vi "Teleop.vi"(10 "Match Info":T1={"Autonomous Elapsed Seconds"=0.0, "TeleOp Elapsed Seconds"=43.06, "Disabled Elapsed Seconds"=6.912, "Visited Autonomous"=FALSE, "Visited TeleOp"=TRUE, "Visited Disabled"=TRUE, "Autonomous Settings"={"Autonomous Style"=enum."Independent", "VI Refnum"=refnum}}, 11 "Call Context":T2=enum."Stop") -> ()   [LabVIEW 2019]
doc: "This VI is called for each TeleOp packet received from the DS where the robot is not disabled. It is often used to read from the joysticks and update I/O or to update setpoints for timed control loops. It should complete and return within 20 milliseconds or it may miss DS packets."
uses:
  <vilib>/Rock Robotics/WPI/DriverStation/WPI_DriverStationDerivedRobotMode.ctl
  <vilib>/Rock Robotics/WPI/DriverStation/WPI_DriverStationMatch Info.ctl
  <vilib>/Rock Robotics/WPI/Solenoid/WPI_SolenoidValue.ctl
  Global Data.vi
  <vilib>/Rock Robotics/Network Tables/NT Write Number.vi
  Refnums.vi
  <vilib>/Rock Robotics/Network Tables/NT Write Numeric Array.vi
  <vilib>/Rock Robotics/Network Tables/NT Write Boolean Array.vi
  Buttons.vi
  <vilib>/Rock Robotics/WPI/Solenoid/WPI_SolenoidSetEnum.vi
  <vilib>/Rock Robotics/WPI/ThirdParty/Phoenix-LabVIEW/Motor Controller/Controls/CTRE_Phoenix_MotorControl_ControlMode.ctl
  <vilib>/Rock Robotics/WPI/ThirdParty/Phoenix-LabVIEW/Motor Controller/Get/CTRE_Phoenix_MotorController_GetQuadratureData.vi
panel:
  in  "f":enum16{"Spin-Up", "Shoot", "Stop"}(ring)
  in  "AngleSet":dbl
  out "Angle Position":dbl=4.0
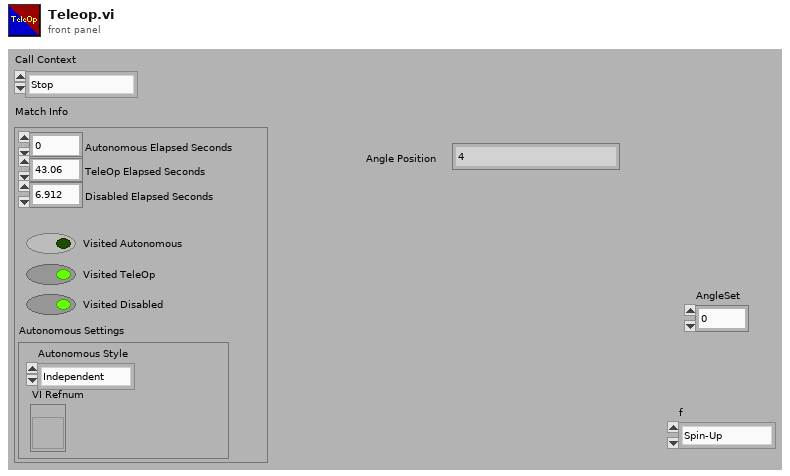
[diagram p1: front panel]
types:
  T1 = typedef "WPI_DriverStationMatch Info.ctl" = cluster{"Autonomous Elapsed Seconds":dbl, "TeleOp Elapsed Seconds":dbl, "Disabled Elapsed Seconds":dbl, "Visited Autonomous":bool, "Visited TeleOp":bool, "Visited Disabled":bool, "Autonomous Settings":cluster{"Autonomous Style":enum16{"Iterative", "Independent"}, "VI Refnum":refnum<vi>}}
  T2 = typedef "WPI_DriverStationDerivedRobotMode.ctl" = enum16{"Init", "Execute", "Stop"}
  T3 = typedef "WPI_SolenoidValue.ctl" = enum16{"Off", "On", "Forward", "Reverse"}
  T4 = typedef "WPI_JoystickDevRef.ctl" = cluster{"Device":T5}
  T5 = typedef "WPI_JoystickDeviceEnum.ctl" = enum16{"USB 0", "USB 1", "USB 2", "USB 3", "USB 4", "USB 5"}
  T6 = cluster{"Align Turret":i32, "Turret Right":i32, "TODO 1":i32, "Turret Left":i32, "Jump Intake":i32, "Shoot":i32, "TODO 2":i32, "TODO 3":i32, "TODO 4":i32, "TODO 5":i32}
  T7 = cluster{"Shift Gear":i32, "Turret Track":i32, "Shoot":i32, "Intake":i32, "Turret Left":i32, "Turret Right":i32, "TODO 2":i32, "TODO 3":i32, "TODO 4":i32, "TODO 5":i32}
  T8 = typedef "CTRE_Phoenix_MotorControl_ControlMode.ctl" = u16
  T9 = typedef "WPI_RobotDriveDevRef.ctl" = cluster{"DevStatus":errorcluster, "Motors[]":T10[], "Square Inputs":bool, "Max Output":dbl}
  T10 = typedef "WPI_MotorControlDeviceRef.ctl" = cluster{"DeviceStatus":errorcluster, "Type":T11, "PWM":cluster{"PWM Channel":T12, "DeadBand":T13}, "CAN":cluster{"Device Number":u8, "SetOutput VI Ref":variant, "GetOutput VI Ref":variant, "Enable VI Ref":variant, "Disable VI Ref":variant, "Data":variant}, "Invert":bool, "DIO PWM":cluster{"PWM \"Enable\" Channel":T12, "DIOChannel":T14, "PWM Rate":dbl}}
  T11 = typedef "WPI_MotorControlType.ctl" = enum16{"PWM", "CAN", "DIO PWM"}
  T12 = typedef "FPGA_DIOPWMChannel.ctl" = enum8{"PWM 0", "PWM 1", "PWM 2", "PWM 3", "PWM 4", "PWM 5", "PWM 6", "PWM 7", "PWM 8", "PWM 9", "PWM MXP 0", "PWM MXP 1", "PWM MXP 2", "PWM MXP 3", "PWM MXP 4", "PWM MXP 5", "PWM MXP 6", "PWM MXP 7", "PWM MXP 8", "PWM MXP 9", "Invalid"}
  T13 = typedef "WPI_PWMDeadband.ctl" = cluster{"Name":string, "maxPositivePwm":i32, "minPositivePwm":i32, "centerPwm":i32, "maxNegativePwm":i32, "minNegativePwm":i32, "angularRange":u16}
  T14 = typedef "FPGA_DIOChannel.ctl" = enum8{"DIO 0", "DIO 1", "DIO 2", "DIO 3", "DIO 4", "DIO 5", "DIO 6", "DIO 7", "DIO 8", "DIO 9", "DIO MXP 0", "DIO MXP 1", "DIO MXP 2", "DIO MXP 3", "DIO MXP 4", "DIO MXP 5", "DIO MXP 6", "DIO MXP 7", "DIO MXP 8", "DIO MXP 9", "DIO MXP 10", "DIO MXP 11", "DIO MXP 12", "DIO MXP 13", "DIO MXP 14", "DIO MXP 15", "SPI Port CS1", "SPI Port CS2", "SPI Port CS3", "SPI Port MISO", "SPI Port MOSI", "Invalid"}
  T15 = cluster{"ROBOT_DRIVE":T9, "TURRET":T10, "SHOOTER_MASTER":T10, "HOPPER":T10, "INDEXER":T10, "INTAKE":T10, "CLIMBER_WINCH":T10, "CLIMBER_ARM":T10, "SHOOTER_ANGLE":T10, "SHOOTER_SLAVE":T10, "AGITATOR":T10, "AGITATOR OLD":T10, "LEFT_MASTER":T10, "RIGHT_MASTER":T10}
  T16 = typedef "WPI_CompressorDevRef.ctl" = cluster{"DevStatus":errorcluster, "Pneumatics Control Module":u8}
  T17 = typedef "WPI_SolenoidDevRef.ctl" = cluster{"DevStatus":errorcluster, "Pneumatics Control Module":u8, "Forward Solenoid Channel":T18, "Reverse Solenoid Channel":T18}
  T18 = typedef "WPI_SolenoidChannel.ctl" = enum8{"Solenoid 0", "Solenoid 1", "Solenoid 2", "Solenoid 3", "Solenoid 4", "Solenoid 5", "Solenoid 6", "Solenoid 7", "Invalid"}
  T19 = cluster{"COMPRESSOR":T16, "SHIFTER":T17, "INTAKE_PIVOT":T17}
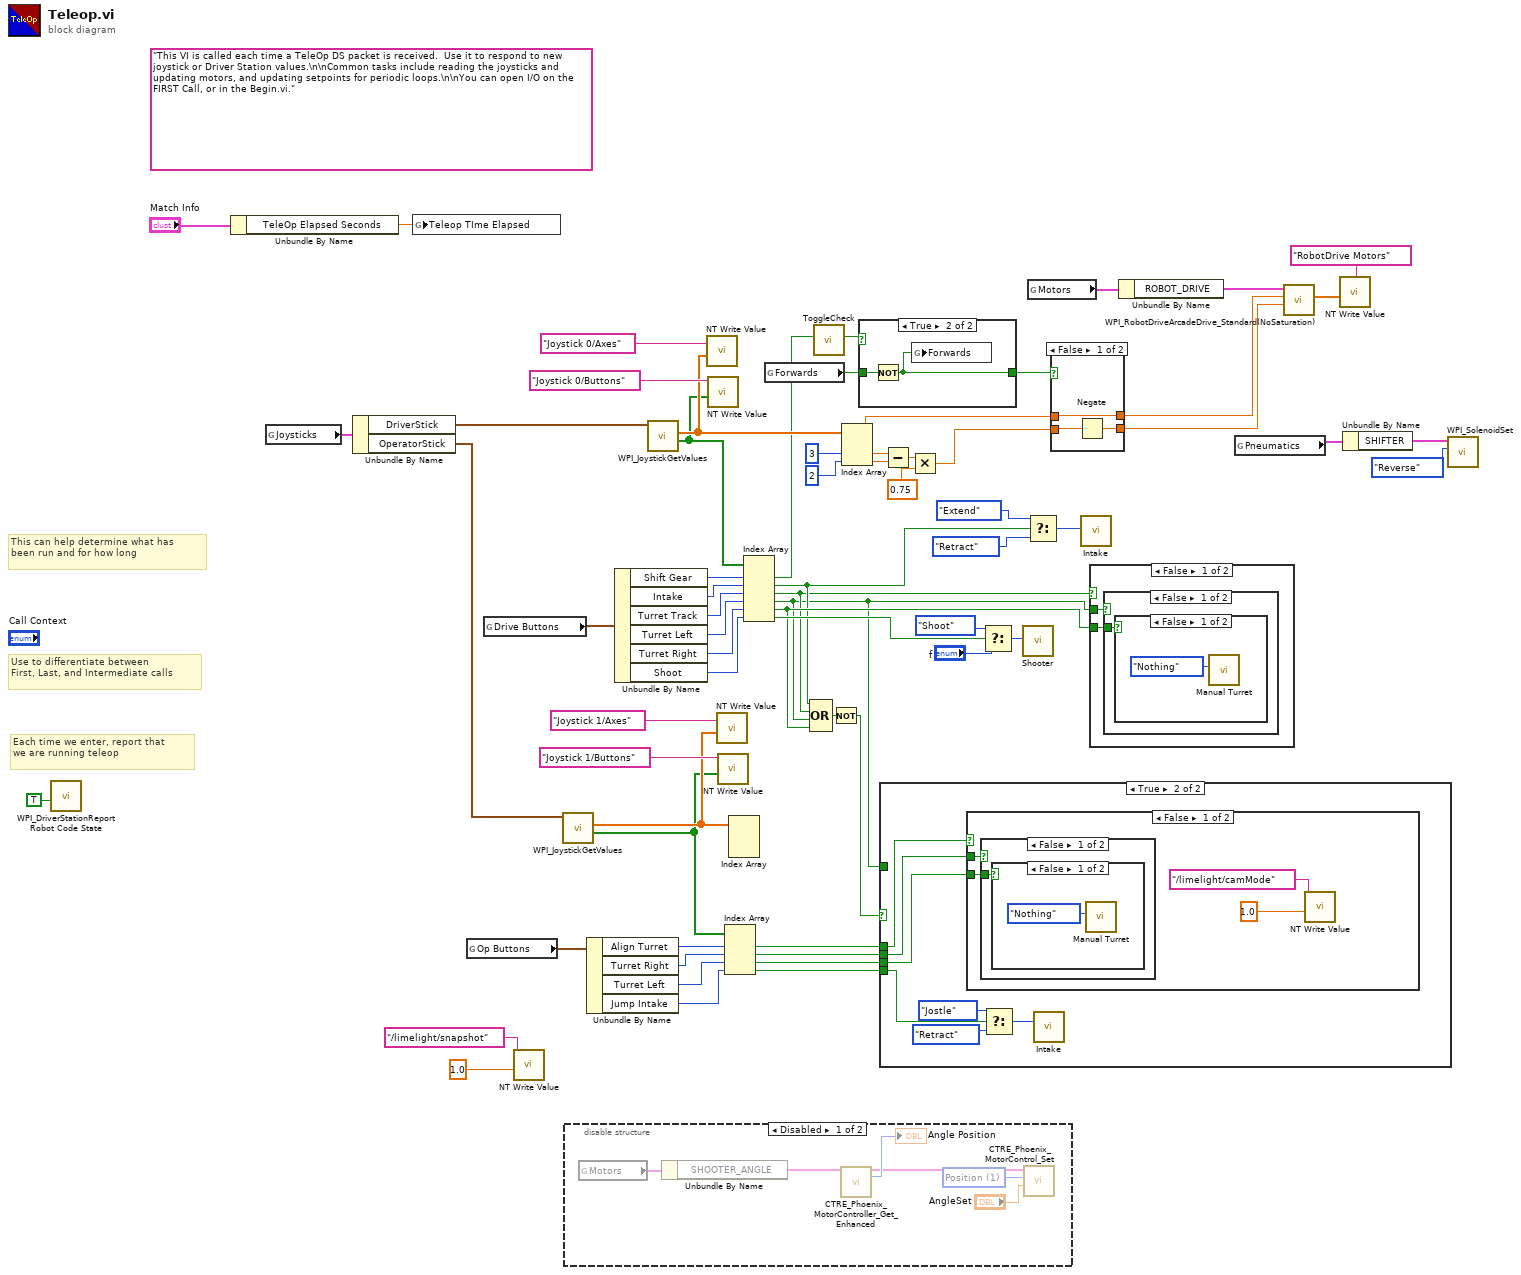
[diagram p0: block diagram]
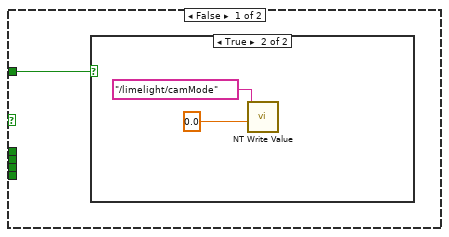
[diagram p2: hidden frame]
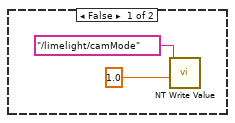
[diagram p3: hidden frame]
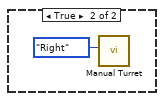
[diagram p4: hidden frame]
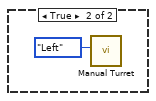
[diagram p5: hidden frame]
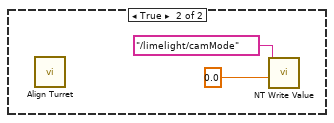
[diagram p6: hidden frame]
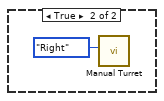
[diagram p10: hidden frame]
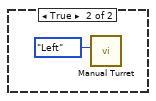
[diagram p11: hidden frame]
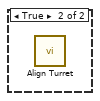
[diagram p12: hidden frame]
diagram:
  (unwired) "This VI is called each time a TeleOp DS packet is received.  Use it to respond to new joystick or Driver Station values.\n\nCommon tasks include reading the joysticks and updating motors, and updating setpoints for periodic loops.\n\nYou can open I/O on the FIRST Call, or in the Begin.vi."
  # "Each time we enter, report that\nwe are running teleop"
  # "Use to differentiate between\nFirst, Last, and Intermediate calls"
  # "This can help determine what has\nbeen run and for how long"
  n1 = call <vilib>:"WPI_DriverStationReport Robot Code State.vi"("TeleOp"=TRUE ("Autonomous")) -> ()  [unwired: 10 in, 1 out]
  n2 = Unbundle By Name("Match Info") -> ("TeleOp Elapsed Seconds"=w44:dbl)
  n3 = global read "Refnums.vi" "Joysticks"() -> (w59:cluster{"DriverStick":T4, "OperatorStick":T4})
  n4 = Unbundle By Name(w59) -> ("DriverStick"=w58:T4, "OperatorStick"=w26:T4)
  n5 = global write "Global Data.vi" "Teleop TIme Elapsed"(w44) -> ()
  n6 = global read "Buttons.vi" "Op Buttons"() -> (w21:T6)
  n7 = global read "Buttons.vi" "Drive Buttons"() -> (w54:T7)
  n8 = call-poly <vilib>:"NT Write Value.vi"("Numeric"=1.0, "Name"="/limelight/snapshot") -> ()  [unwired: 9 in, 1 out]
  n9 = call <vilib>:"WPI_JoystickGetValues.vi"("JoystickDevRef"=w26) -> ("Buttons"=w22:bool[], "Axes"=w23:dbl[])  [unwired: 6 in, 3 out]
  n10 = disable-structure shown="Disabled" {
    frame Disabled {
      w68 = T8 1 items=["PercentOutput"=0, "Position"=1, "Velocity"=2, "Current"=3, "Follower"=5, "MotionProfile"=6, "MotionMagic"=7, "MotionProfileArc"=10, "Disabled"=15] ("Control Mode")
      n11 = global read "Refnums.vi" "Motors"() -> (w72:T15)
      n12 = Unbundle By Name(w72) -> ("SHOOTER_ANGLE"=w69:T10)
      n13 = call-poly <vilib>:"CTRE_Phoenix_MotorController_Get_Enhanced.vi"("PhoenixMotorControlDevRef"=w69) -> ("PhoenixMotorControlDevRef"=w70:T10, "Quadrature Position"=→"Angle Position":i32)  [unwired: 11 in, 2 out]
      n14 = call <vilib>:"CTRE_Phoenix_MotorControl_Set.vi"("Output"="AngleSet", "Control Mode"=w68, "PhoenixMotorControlDevRef"=w70) -> ()  [unwired: 7 in, 2 out]
    }
    frame Enabled {
    }
  }
  n15 = Unbundle By Name(w21) -> ("Align Turret"=w20:i32, "Turret Right"=w8:i32, "Turret Left"=w9:i32, "Jump Intake"=w10:i32)
  n16 = Unbundle By Name(w54) -> ("Shift Gear"=w53:i32, "Intake"=w52:i32, "Turret Track"=w51:i32, "Turret Left"=w50:i32, "Turret Right"=w49:i32, "Shoot"=w48:i32)
  n17 = call <vilib>:"WPI_JoystickGetValues.vi"("JoystickDevRef"=w58) -> ("Buttons"=w55:bool[], "Axes"=w62:dbl[])  [unwired: 6 in, 3 out]
  n18 = call-poly <vilib>:"NT Write Value.vi"("Numeric Array"=w62, "Name"="Joystick 0/Axes") -> ()  [unwired: 9 in, 1 out]
  n19 = call-poly <vilib>:"NT Write Value.vi"("Boolean Array"=w55, "Name"="Joystick 0/Buttons") -> ()  [unwired: 9 in, 1 out]
  n20 = call-poly <vilib>:"NT Write Value.vi"("Numeric Array"=w23, "Name"="Joystick 1/Axes") -> ()  [unwired: 9 in, 1 out]
  n21 = call-poly <vilib>:"NT Write Value.vi"("Boolean Array"=w22, "Name"="Joystick 1/Buttons") -> ()  [unwired: 9 in, 1 out]
  n22 = Index Array(array=w22, index #1=w20, index #2=w8, index #3=w9, index #4=w10) -> (element #1=w14:bool, element #2=w13:bool, element #3=w12:bool, element #4=w11:bool)
  n23 = Index Array(array=w23) -> ()  [unwired: 3 in, 3 out]
  n24 = Index Array(array=w55, index #1=w53, index #2=w52, index #3=w51, index #4=w50, index #5=w49, index #6=w48) -> (element #1=w38:bool, element #2=w15:bool, element #3=w4:bool, element #4=w3:bool, element #5=w18:bool, element #6=w19:bool)
  n25 = global read "Global Data.vi" "Forwards"() -> (w31:bool)
  n26 = Compound Arithmetic op=OR(w15, w4, w3, w18) -> (w17:bool)
  n27 = call "ToggleCheck.vi"("button in"=w38) -> ("toggled?"=w32:bool)  [unwired: 10 in]
  n28 = Not(x=w17) -> (.not. x?=w16:bool)
  n29 = Index Array(array=w62, index #2=3 ("index"), index #3=2 ("index")) -> (element #1=w37:dbl, element #2=w41:dbl, element #3=w40:dbl)  [unwired: 1 in]
  n30 = case shown="True" w32 {
    tunnel: w31 -> [w73 w75]
    tunnel: [w73 w74] -> w30
    frame False {
    }
    frame True {
      n31 = Not(x=w75) -> (.not. x?=w74:bool)
      n32 = global write "Global Data.vi" "Forwards"(w74) -> ()
    }
  }
  n33 = case shown="True" w16 {
    tunnel: w14 -> [_ w83]
    tunnel: w13 -> [_ w82]
    tunnel: w12 -> [_ w81]
    tunnel: w11 -> [_ w85]
    tunnel: w3 -> [w76 _]
    frame False {
      n34 = case shown="True" w76 {
        frame False {
          n35 = call-poly <vilib>:"NT Write Value.vi"("Numeric"=1.0, "Name"="/limelight/camMode") -> ()  [unwired: 9 in, 1 out]
        }
        frame True {
          n36 = call-poly <vilib>:"NT Write Value.vi"("Numeric"=0.0, "Name"="/limelight/camMode") -> ()  [unwired: 9 in, 1 out]
        }
      }
    }
    frame True {
      n37 = case shown="False" w83 {
        tunnel: w82 -> [w91 _]
        tunnel: w81 -> [w90 _]
        frame False {
          n38 = case shown="False" w91 {
            tunnel: w90 -> [w92 _]
            frame False {
              n39 = case shown="False" w92 {
                frame False {
                  n40 = call "Manual Turret.vi"("Enum"=enum16{"Nothing", "Left", "Right"}."Nothing") -> ()  [unwired: 11 in]
                }
                frame True {
                  n41 = call "Manual Turret.vi"("Enum"=enum16{"Nothing", "Left", "Right"}."Right") -> ()  [unwired: 11 in]
                }
              }
            }
            frame True {
              n42 = call "Manual Turret.vi"("Enum"=enum16{"Nothing", "Left", "Right"}."Left") -> ()  [unwired: 11 in]
            }
          }
          n43 = call-poly <vilib>:"NT Write Value.vi"("Numeric"=1.0, "Name"="/limelight/camMode") -> ()  [unwired: 9 in, 1 out]
        }
        frame True {
          n44 = call "Align Turret.vi"() -> ()  [unwired: 12 in]
          n45 = call-poly <vilib>:"NT Write Value.vi"("Numeric"=0.0, "Name"="/limelight/camMode") -> ()  [unwired: 9 in, 1 out]
        }
      }
      n46 = Select(t=enum16{"Retract", "Jostle", "Extend"}."Jostle" ("Enum"), s=w85, f=enum16{"Retract", "Jostle", "Extend"}."Retract" ("Enum")) -> (s? t:f=w84:enum16{"Retract", "Jostle", "Extend"})
      n47 = call "Intake.vi"("Enum"=w84) -> ()  [unwired: 11 in]
    }
  }
  n48 = Subtract(x=w41, y=w40) -> (x-y=w34:dbl)
  n49 = Multiply(x=w34, y=0.75) -> (x*y=w35:dbl)
  n50 = Select(t=enum16{"Spin-Up", "Shoot", "Stop"}."Shoot" ("Action"), s=w19, f="f") -> (s? t:f=w46:enum16{"Spin-Up", "Shoot", "Stop"})
  n51 = call "Shooter.vi"("Action"=w46) -> ()  [unwired: 11 in]
  n52 = global read "Refnums.vi" "Motors"() -> (w57:T15)
  n53 = Select(t=enum16{"Retract", "Jostle", "Extend"}."Extend" ("Enum"), s=w15, f=enum16{"Retract", "Jostle", "Extend"}."Retract" ("Enum")) -> (s? t:f=w5:enum16{"Retract", "Jostle", "Extend"})
  n54 = case shown="False" w30 {
    tunnel: [w100 w101] -> w39
    tunnel: w35 -> [w99 w101]
    tunnel: [w98 w102] -> w36
    tunnel: w37 -> [w98 w102]
    frame False {
      n55 = Negate(x=w99) -> (-x=w100:dbl)
    }
    frame True {
    }
  }
  n56 = call "Intake.vi"("Enum"=w5) -> ()  [unwired: 11 in]
  n57 = case shown="False" w4 {
    tunnel: w3 -> [w104 _]
    tunnel: w18 -> [w103 _]
    frame False {
      n58 = case shown="False" w104 {
        tunnel: w103 -> [w105 _]
        frame False {
          n59 = case shown="False" w105 {
            frame False {
              n60 = call "Manual Turret.vi"("Enum"=enum16{"Nothing", "Left", "Right"}."Nothing") -> ()  [unwired: 11 in]
            }
            frame True {
              n61 = call "Manual Turret.vi"("Enum"=enum16{"Nothing", "Left", "Right"}."Right") -> ()  [unwired: 11 in]
            }
          }
        }
        frame True {
          n62 = call "Manual Turret.vi"("Enum"=enum16{"Nothing", "Left", "Right"}."Left") -> ()  [unwired: 11 in]
        }
      }
    }
    frame True {
      n63 = call "Align Turret.vi"() -> ()  [unwired: 12 in]
    }
  }
  n64 = Unbundle By Name(w57) -> ("ROBOT_DRIVE"=w56:T9)
  n65 = global read "Refnums.vi" "Pneumatics"() -> (w29:T19)
  n66 = call <vilib>:"WPI_RobotDriveArcadeDrive_Standard(NoSaturation).vi"("Y axis value"=w39, "X axis value"=w36, "RobotDriveDevRef"=w56) -> ("Motor Values"=w61:dbl[])  [unwired: 1 in, 7 out]
  n67 = call-poly <vilib>:"NT Write Value.vi"("Numeric Array"=w61, "Name"="RobotDrive Motors") -> ()  [unwired: 9 in, 1 out]
  n68 = Unbundle By Name(w29) -> ("SHIFTER"=w28:T17)
  n69 = call-poly <vilib>:"WPI_SolenoidSet.vi"("Value"=WPI_SolenoidValue."Reverse", "SolenoidDevRef"=w28) -> ()  [unwired: 8 in, 2 out]
